vi "Auto Ring_recipe.vi"(8 "error in (no error)":errorcluster, 11 "Master in":refnum<class "Master.lvclass">) -> (0 "error out":errorcluster, 3 "Master out":refnum<class "Master.lvclass">, 4 "Array":string[](array[string]), 6 "Array 2":string[][](array[string]))   [LabVIEW 2014, in "Master.lvclass"]
uses:
  Master/Master.lvclass
  Master/Master.lvclass/Master.ctl
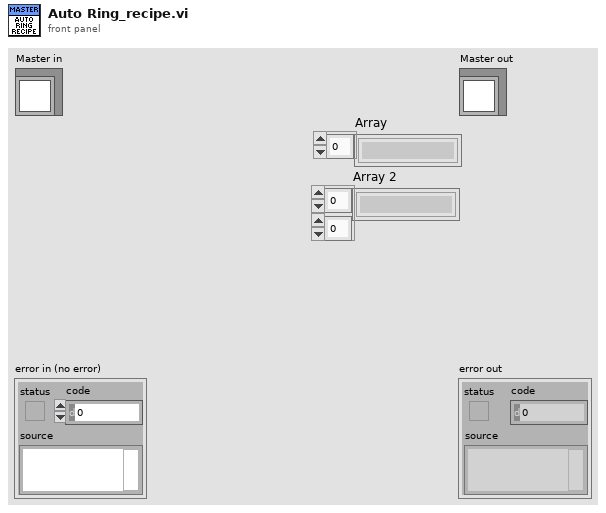
[diagram p1: front panel]
types:
  T1 = cluster{"Name":string, "Wind Length":string, "Wind Spd":string, "Kink Cyc":string, "Bind Length":string, "Unit":string}[]
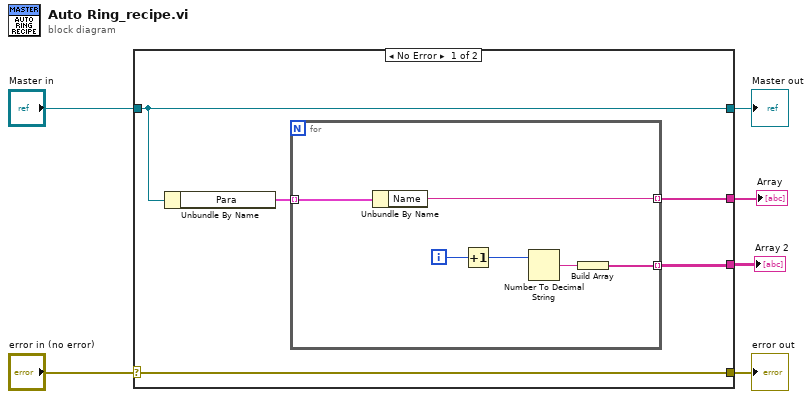
[diagram p0: block diagram]
diagram:
  n1 = case shown="No Error" "error in (no error)" {
    selector: "error in (no error)" -> [w11 w19]
    tunnel: [w11 w19] -> w5
    tunnel: [w10 w18] -> w3
    tunnel: "Master in" -> [w10 w18]
    tunnel: [w8 _] -> w2
    tunnel: [w7 _] -> w1
    frame No Error {
      n2 = Unbundle By Name(w10) -> ("Para"=w9:T1)
      n3 = for {
        tunnel: w9 -> [w17] mode=indexing
        tunnel: [w16] -> w8 mode=indexing
        tunnel: [w12] -> w7 mode=indexing
        i -> [w15]
        n4 = Unbundle By Name(w17) -> ("Name"=w16:string)
        n5 = Increment(x=w15) -> (x+1=w13:i32)
        n6 = Number To Decimal String(number=w13) -> (decimal integer string=w14:string)  [unwired: 1 in]
        n7 = Build Array(w14) -> (w12:string[])
      }
    }
    frame Error {
    }
  }
  "error out" <- w5
  "Master out" <- w3
  "Array" <- w2
  "Array 2" <- w1
